vi "Keep position above object.vi"(7 "Numeric":dbl, 8 "bottom":dbl, 9 "right":dbl, 10 "top":dbl, 11 "left":dbl) -> (0 "Hover":bool, 1 "Roll":dbl, 2 "Pitch":dbl)   [LabVIEW 2014]
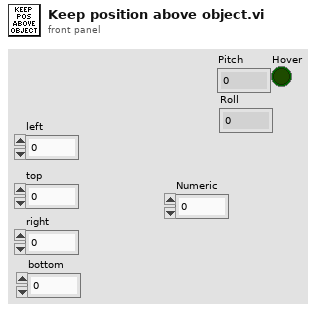
[diagram p1: front panel]
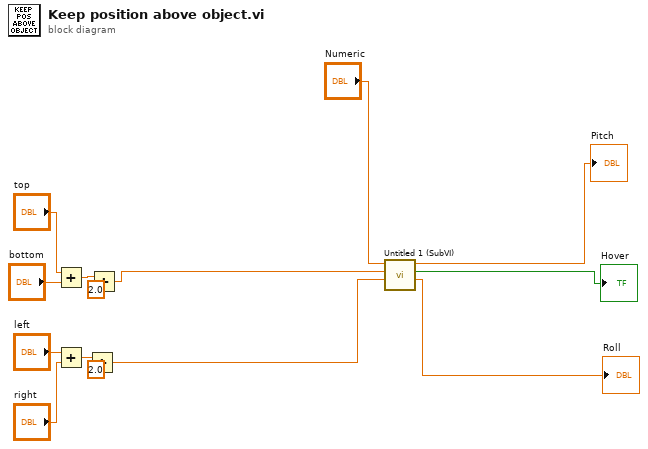
[diagram p0: block diagram]
diagram:
  n1 = Add(x="top", y="bottom") -> (x+y=w8:dbl)
  n2 = Add(x="left", y="right") -> (x+y=w7:dbl)
  n3 = Divide(x=w7, y=2.0) -> (x/y=w5:dbl)
  n4 = Divide(x=w8, y=2.0) -> (x/y=w6:dbl)
  n5 = call "Untitled 1 (SubVI).vi"("Numeric 2"=w5, "Numeric 3"=w6, "Numeric"="Numeric") -> ("Roll"=→"Roll":dbl, "Hover"=→"Hover":bool, "Pitch"=→"Pitch":dbl)  [unwired: 6 in]
